vi "LDR M U for integrated.vi"(0 "LINX Resource 2":T1, 2 "Knob":dbl(knob) scale=0.0..1.0, 3 "Echo":u8, 7 "LDR Analog pin":u8, 10 "Trigger":u8, 11 "Enable PWM Channel for  motor":u8, 14 "IN2 Motor":u8, 15 "stop of ldr while":bool, 20 "Error Out 2":errorcluster) -> (1 "Light Intensity":dbl, 4 "voltage across ldr":dbl, 6 "LINX Resource":T1, 8 "U1 Distance(cm)":u32, 12 "Pulse Width (uS)":u32, 26 "Waveform Chart u1":dbl(graph))   [LabVIEW 2020]
uses:
  <vilib>/MakerHub/LINX/Private/Type Defs/LINX Ref.ctl
  <vilib>/MakerHub/LINX/Private/Type Defs/Platform.ctl
  <vilib>/MakerHub/LINX/Private/Type Defs/Interface.ctl
  <vilib>/MakerHub/LINX/Private/Device/Type Defs/LINX Device Config.ctl
  <vilib>/MakerHub/LINX/Private/Device/Type Defs/TCP Config.ctl
  <vilib>/MakerHub/LINX/Private/Device/Type Defs/Channels.ctl
  <vilib>/MakerHub/LINX/Private/Device/Type Defs/Stimulus Pulse.ctl
  <vilib>/MakerHub/LINX/Public/Peripherals/Analog/Analog Read 1 Chan.vi
  <vilib>/MakerHub/LINX/Public/Peripherals/Digital/Digital Write 1 Chan.vi
  <vilib>/MakerHub/LINX/Public/Peripherals/PWM/PWM Set Duty Cycle 1 Chan.vi
  <vilib>/MakerHub/LINX/Public/Peripherals/Analog/Analog Read N Chans.vi
  <vilib>/MakerHub/LINX/Public/Peripherals/Digital/Digital Write N Chans.vi
  <vilib>/MakerHub/LINX/Private/Local IO/LinxAnalogRead.vi
  <vilib>/MakerHub/LINX/Public/Utilities/Check Channel.vi
  <vilib>/MakerHub/LINX/Private/Local IO/LinxDigitalWrite.vi
  <vilib>/MakerHub/LINX/Private/Utilties/Generate Error.vi
  <vilib>/MakerHub/LINX/Public/Peripherals/PWM/PWM Set Duty Cycle N Chans.vi
  <vilib>/MakerHub/LINX/Private/Device/Device.lvlib
  <vilib>/MakerHub/LINX/LMH-LINX.lvlib
panel:
  in  "IN1 Motor":u8
  out "Waveform Chart u1\n 2":dbl(graph)
  out "U1 Distance(cm) 2":u32
  out "Pulse Width (uS) 2":u32
  in  "Echo 2":u8
  in  "Trigger 2":u8
  out "Error Out":errorcluster
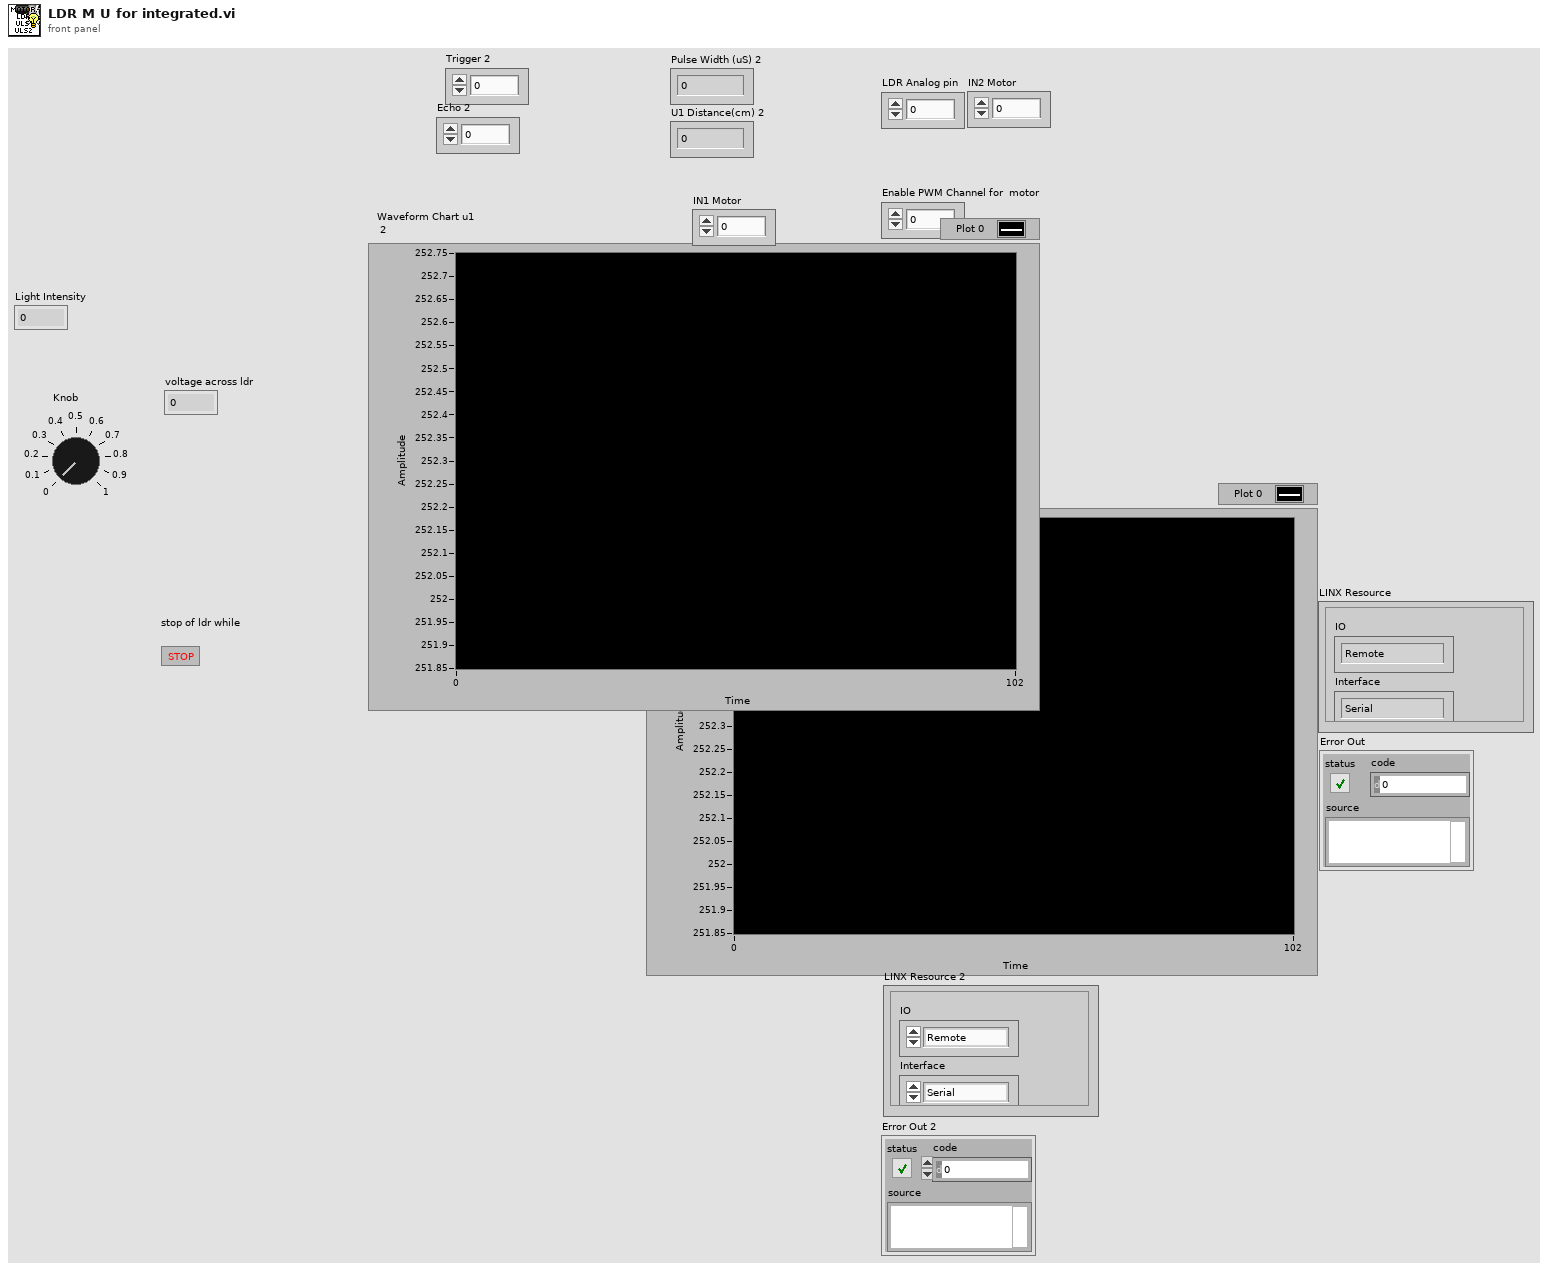
[diagram p1: front panel]
types:
  T1 = typedef "LMH-LINX.lvlib/LINX Ref.ctl" = cluster{"IO":T2, "Interface":T3, "LINX Device Config":T4}
  T2 = typedef "LMH-LINX.lvlib/Platform.ctl" = enum16{"Remote", "Local"}
  T3 = typedef "LMH-LINX.lvlib/Interface.ctl" = enum16{"Serial", "TCP"}
  T4 = typedef "LMH-LINX.lvlib/Device.lvlib/LINX Device Config.ctl" = cluster{"Interface":T3, "COM Port":refnum<visa-resource-name>, "TCP Configuration":T5, "Device Family":u8, "Device ID":u8, "Device Name":string, "TCP Ref":refnum<k5>, "Channels":T6}
  T5 = typedef "LMH-LINX.lvlib/Device.lvlib/TCP Config.ctl" = cluster{"IP Address":string, "Port":u16}
  T6 = typedef "LMH-LINX.lvlib/Channels.ctl" = cluster{"DI":u8[], "DO":u8[], "AI":u8[], "AO":u8[], "PWM":u8[], "QE":u8[], "UART":u8[], "I2C 2":u8[], "SPI":u8[], "CAN":u8[], "Servo":u8[], "AI Ref (V)":dbl, "AI Resolution (Bits)":u8, "AO Ref (V)":dbl, "AO Resolution (Bits)":u8}
  T7 = typedef "LMH-LINX.lvlib/Device.lvlib/Stimulus Pulse.ctl" = enum16{"None", "Active Low", "Active High"}
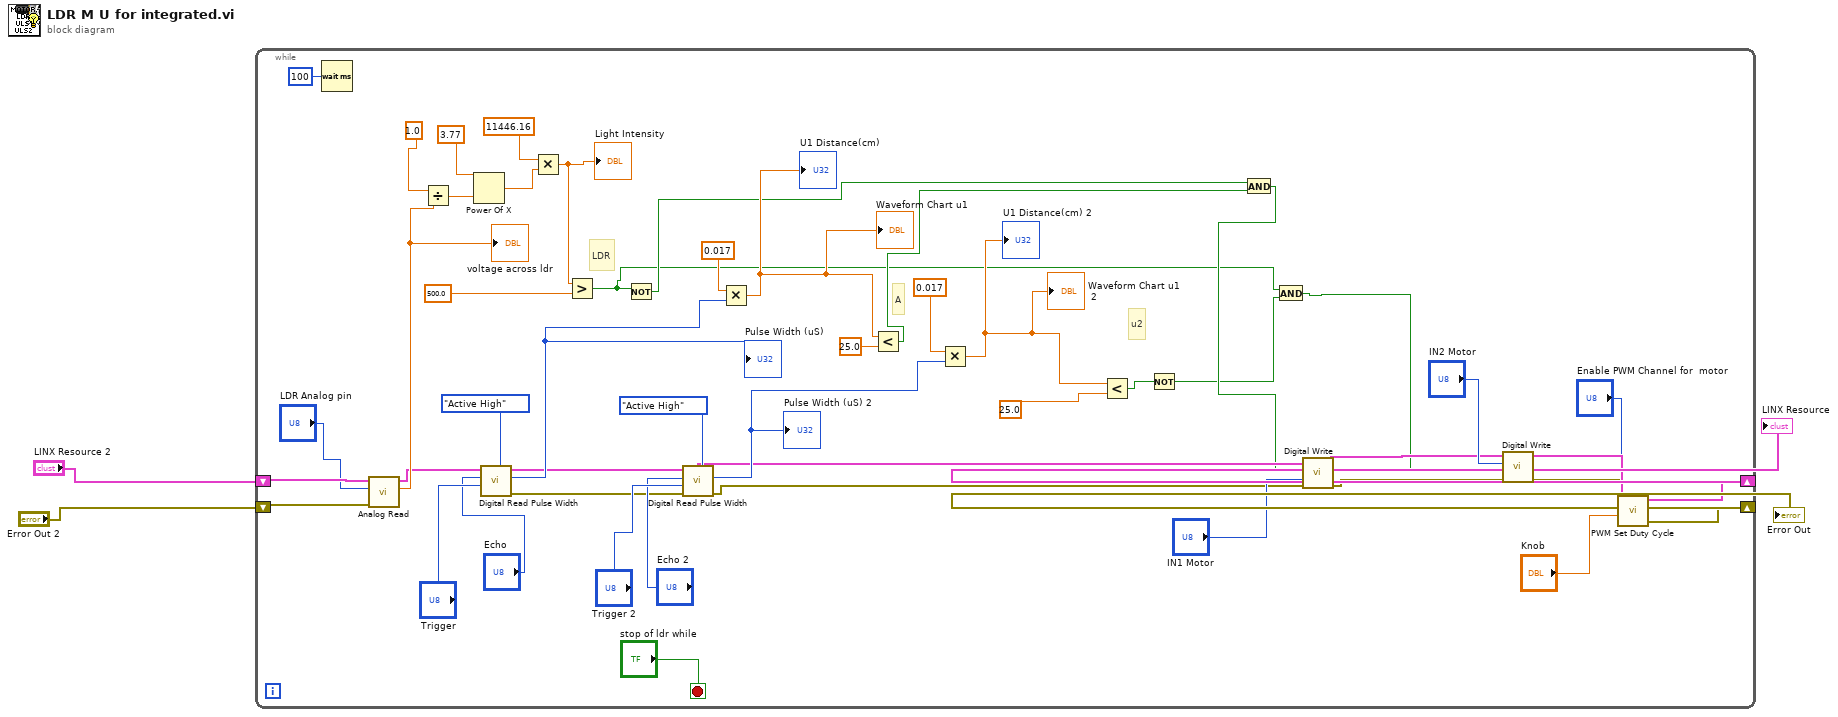
[diagram p0: block diagram]
diagram:
  n1 = while {
    shift-right: [w33] -> w4
    shift-left: "LINX Resource 2" -> [w53]
    shift-right: [w32] -> w3
    shift-left: "Error Out 2" -> [w52]
    stop <- "stop of ldr while" stop-if-true
    # "u2"
    # "A"
    # "LDR"
    n2 = Wait (ms)(milliseconds to wait=u32 100) -> ()  [unwired: 1 out]
    n3 = call-poly <vilib>:"Analog Read.vi"("Error In"=w52, "Analog Channel"="LDR Analog pin", "LINX Resource"=w53) -> ("Voltage"=w44:dbl, "LINX Resource"=w31:T1)  [unwired: 5 in, 2 out]
    "voltage across ldr" <- w44
    n4 = Divide(x=1.0, y=w44) -> (x/y=w48:dbl)
    n5 = Power Of X(1:w48, 2:3.77 ("y")) -> (0:w46:dbl)
    n6 = call <vilib>:"Digital Read Pulse Width.vi"("Stimulus Pulse (Active High)"=Stimulus_Pulse."Active High", "DO Channel"="Trigger", "DI Channel"="Echo", "LINX Resource"=w31) -> ("Error Out"=w16:errorcluster, "Pulse Width (uS)"=w38:u32, "LINX Resource"=w17:T1)  [unwired: 5 in]
    "Pulse Width (uS)" <- w38
    n7 = Multiply(x=11446.16, y=w46) -> (x*y=w30:dbl)
    "Light Intensity" <- w30
    n8 = Greater?(x=w30, y=500.0) -> (0:w6:bool)
    n9 = Not(x=w6) -> (.not. x?=w11:bool)
    n10 = call <vilib>:"Digital Read Pulse Width.vi"("Stimulus Pulse (Active High)"=Stimulus_Pulse."Active High", "Error In"=w16, "DO Channel"="Trigger 2", "DI Channel"="Echo 2", "LINX Resource"=w17) -> ("Error Out"=w14:errorcluster, "Pulse Width (uS)"=w19:u32, "LINX Resource"=w15:T1)  [unwired: 4 in]
    "Pulse Width (uS) 2" <- w19
    n11 = Multiply(x=0.017, y=w38) -> (x*y=w37:dbl)
    "U1 Distance(cm)" <- w37
    "Waveform Chart u1" <- w37
    n12 = Less?(x=w37, y=25.0) -> (x < y?=w10:bool)
    n13 = Multiply(x=0.017, y=w19) -> (x*y=w21:dbl)
    "U1 Distance(cm) 2" <- w21
    "Waveform Chart u1\n 2" <- w21
    n14 = Less?(x=w21, y=25.0) -> (x < y?=w7:bool)
    n15 = Not(x=w7) -> (.not. x?=w5:bool)
    n16 = And(x=w11, y=w10) -> (x .and. y?=w9:bool)
    n17 = And(x=w6, y=w5) -> (x .and. y?=w8:bool)
    n18 = call-poly <vilib>:"Digital Write.vi"("Error In"=w14, "Output Value"=w9, "DO Channel"="IN1 Motor", "LINX Resource"=w15) -> ("Error Out"=w12:errorcluster, "LINX Resource"=w13:T1)  [unwired: 6 in]
    n19 = call-poly <vilib>:"Digital Write.vi"("Error In"=w12, "Output Value"=w8, "DO Channel"="IN2 Motor", "LINX Resource"=w13) -> ("Error Out"=w42:errorcluster, "LINX Resource"=w43:T1)  [unwired: 6 in]
    n20 = call-poly <vilib>:"PWM Set Duty Cycle.vi"("Error In"=w42, "Duty Cycle (0-1)"="Knob", "PWM Channel"="Enable PWM Channel for  motor", "LINX Resource"=w43) -> ("Error Out"=w32:errorcluster, "LINX Resource"=w33:T1)  [unwired: 6 in]
  }
  "LINX Resource" <- w4
  "Error Out" <- w3
